vi "Projectile.vi"(0 "v (m/s)":dbl, 1 "Theta (deg)":dbl) -> (2 "Max. Height (m)":dbl format="%.3f", 3 "Time of Flight (sec)":dbl format="%.3f", 4 "Range (m)":dbl format="%.3f")   [LabVIEW 2015]
doc: "This is a vi program which can be used as Sub-VI to calculate Maximum Height, Time of Flight and Range of a projectile with given initial velocity and projection angle."
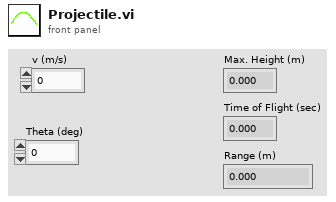
[diagram p1: front panel]
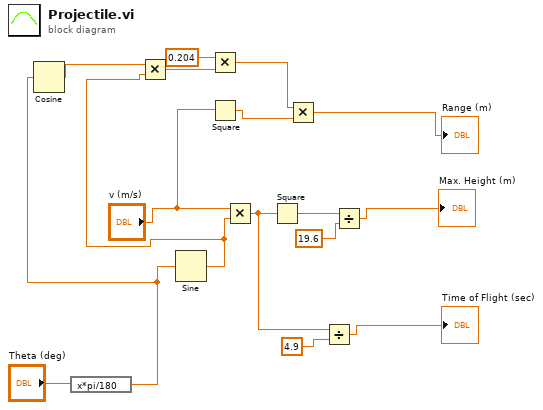
[diagram p0: block diagram]
diagram:
  n1 = expression code="x*pi/180"("Theta (deg)") -> (w1:dbl)
  n2 = Cosine(x=w1) -> (cos(x)=w8:dbl)
  n3 = Sine(x=w1) -> (sin(x)=w7:dbl)
  n4 = Multiply(x=w8, y=w7) -> (x*y=w6:dbl)
  n5 = Multiply(x=0.204, y=w6) -> (x*y=w4:dbl)
  n6 = Square(x="v (m/s)") -> (x^2=w9:dbl)
  n7 = Multiply(x="v (m/s)", y=w7) -> (x*y=w13:dbl)
  n8 = Square(x=w13) -> (x^2=w16:dbl)
  n9 = Multiply(x=w4, y=w9) -> (x*y=→"Range (m)":dbl)
  n10 = Divide(x=w13, y=4.9) -> (x/y=→"Time of Flight (sec)":dbl)
  n11 = Divide(x=w16, y=19.6) -> (x/y=→"Max. Height (m)":dbl)
